vi "TcA01-007_ObjectsCanBeLookedUpByName.vi"(1 "Input buffer":T3="1", 3 "Invocation info":T2, 5 "error in (no error)":errorcluster, 6 "Add log to result?":bool) -> (16 "Test Data":T1 {"Numeric Measurement" format="%.2f"}, 19 "error out":errorcluster)   [LabVIEW 2020]
doc: "Test case template."
uses:
  Shared/Support_InputBuffer.ctl
  Shared/Support_InvocationInfo.ctl
  Shared/Support_TestData.ctl
  <vilib>/addons/_AddQ/G#Object/utils/G#Object_CreateMethod.ctl
  TestClasses/G#BaseClass1_class/G#BaseClass1.lvclass
  TestClasses/G#SubClass1_class/G#SubClass1.lvclass
  <vilib>/addons/_AddQ/G#Object/G#Object.lvclass
panel:
  in  "Test name":string="TcA01-007 Objects can be looked up by name"
  out "Test result":bool
  out "Result":string
  # "Verify that objects can be looked up by name and\nreturn that objects reference instead."
  # "Sub test case"
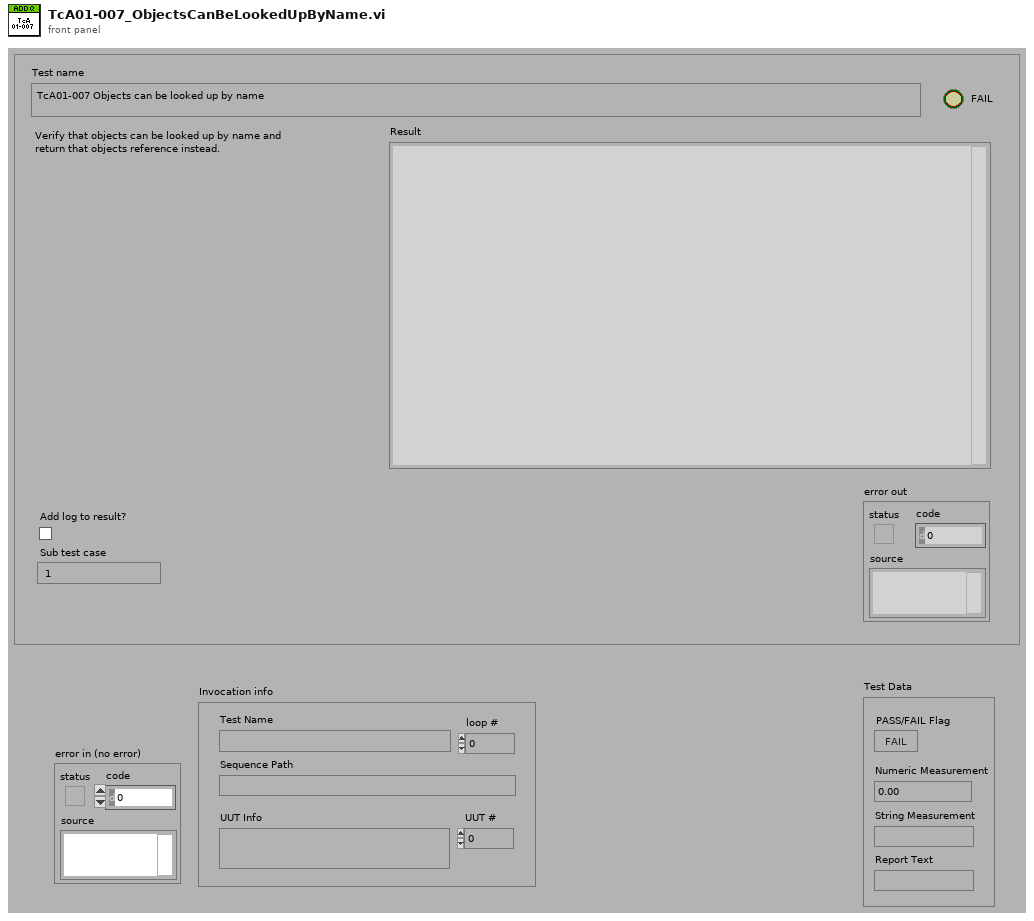
[diagram p1: front panel]
types:
  T1 = typedef "Support_TestData.ctl" = cluster{"PASS/FAIL Flag":bool, "Numeric Measurement":dbl, "String Measurement":string, "Report Text":string}
  T2 = typedef "Support_InvocationInfo.ctl" = cluster{"UUT #":i32, "loop #":i32, "UUT Info":string, "Test Name":string, "Sequence Path":path}
  T3 = typedef "Support_InputBuffer.ctl" = string
  T4 = typedef "G#Object.lvclass/G#Object_CreateMethod.ctl" = enum16{"Create", "Create or look up existing", "Look up existing"}
  T5 = typedef "Support_ResultType.ctl" = cluster{"Pass":bool, "Comment":string, "MeasurementValue":dbl}
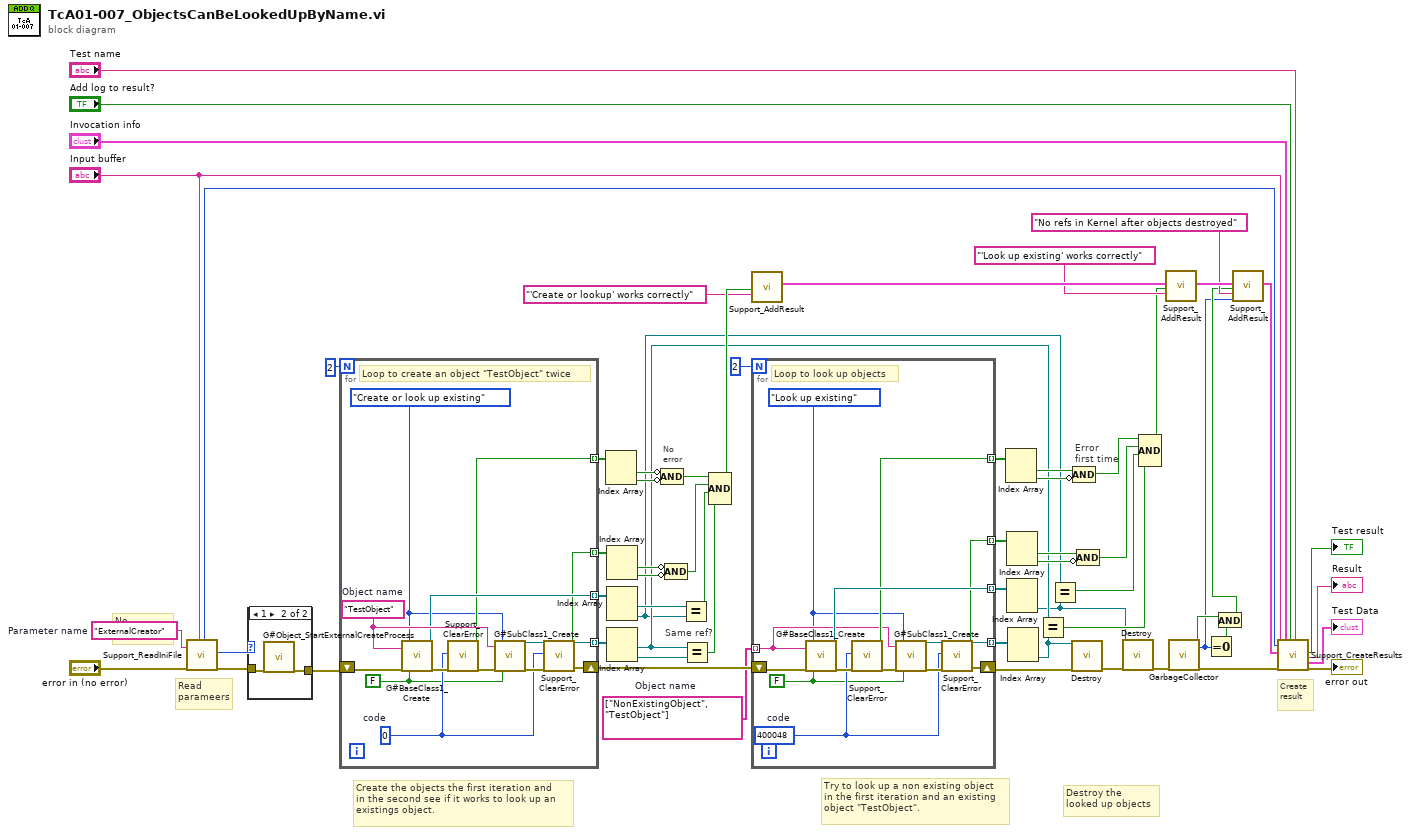
[diagram p0: block diagram]
diagram:
  w3 = "ExternalCreator"  # Parameter name
  w30 = string[] ["NonExistingObject", "TestObject"]  # Object name
  # "Create the objects the first iteration and\nin the second see if it works to look up an\nexistings object."
  # "Try to look up a non existing object\nin the first iteration and an existing\nobject \"TestObject\"."
  # "Destroy the\nlooked up objects"
  # "Error\nfirst time"
  # "Same ref?"
  # "No\nerror"
  # "No\nparameters"
  # "Create\nresult"
  # "Read\nparameers"
  n1 = call "Support_ReadIniFile.vi"("Parameter name"=w3, "error in (no error)"="error in (no error)", "Sub test case"="Input buffer") -> ("Timer start"=w55:u32, "Parameter1 as I32"=w5:i32, "error out"=w6:errorcluster)  [unwired: 9 in, 5 out]
  n2 = case shown="1" w5 {
    tunnel: w6 -> [w65 w67]
    tunnel: [w65 w66] -> w4
    frame 0, Default {
    }
    frame 1 {
      n3 = call <vilib>:"G#Object_StartExternalCreateProcess.vi"("error in (no error)"=w67) -> ("error out"=w66:errorcluster)  [unwired: 18 in]
    }
  }
  n4 = for {
    N: 2 -> [_]
    shift-right: [w72] -> w32
    shift-left: w4 -> [w77]
    tunnel: [w75] -> w51 mode=indexing
    tunnel: [w74] -> w50 mode=indexing
    tunnel: [w71] -> w53 mode=indexing
    tunnel: [w70] -> w52 mode=indexing
    w68 = FALSE ("user counter")
    w69 = G#Object_CreateMethod."Create or look up existing" ("create method")
    w73 = 0  # code
    w76 = "TestObject"  # Object name
    # "Loop to create an object \"TestObject\" twice"
    n5 = call "G#BaseClass1_Create.vi"("object name"=w76, "error in (no error)"=w77, "create method"=w69, "user counter"=w68) -> ("reference out"=w75:refnum<class "G#BaseClass1.lvclass">, "error out"=w78:errorcluster)  [unwired: 13 in, 1 out]
    n6 = call "Support_ClearError.vi"("code"=w73, "error in (no error)"=w78) -> ("Cleared?"=w71:bool, "error out"=w79:errorcluster)  [unwired: 16 in]
    n7 = call "G#SubClass1_Create.vi"("object name"=w76, "error in (no error)"=w79, "create method"=w69, "user counter"=w68) -> ("reference out"=w74:refnum<class "G#SubClass1.lvclass">, "error out"=w80:errorcluster)  [unwired: 13 in, 1 out]
    n8 = call "Support_ClearError.vi"("code"=w73, "error in (no error)"=w80) -> ("Cleared?"=w70:bool, "error out"=w72:errorcluster)  [unwired: 16 in]
  }
  n9 = Index Array(array=w53) -> (element #1=w47:bool, element #2=w46:bool)  [unwired: 2 in]
  n10 = Index Array(array=w52) -> (element #1=w45:bool, element #2=w44:bool)  [unwired: 2 in]
  n11 = Index Array(array=w51) -> (element #1=w49:refnum<class "G#BaseClass1.lvclass">, element #2=w2:refnum<class "G#BaseClass1.lvclass">)  [unwired: 2 in]
  n12 = Index Array(array=w50) -> (element #1=w13:refnum<class "G#SubClass1.lvclass">, element #2=w48:refnum<class "G#SubClass1.lvclass">)  [unwired: 2 in]
  n13 = Compound Arithmetic op=AND(invert w47, invert w46) -> (w43:bool)
  n14 = Compound Arithmetic op=AND(invert w45, invert w44) -> (w42:bool)
  n15 = Equal?(x=w49, y=w2) -> (x = y?=w41:bool)
  n16 = Equal?(x=w13, y=w48) -> (x = y?=w40:bool)
  n17 = Compound Arithmetic op=AND(w43, w42, w41, w40) -> (w39:bool)
  n18 = call "Support_AddResult.vi"("Pass"=w39, "Comment"="'Create or lookup' works correctly") -> ("Results out"=w37:T5[])  [unwired: 17 in]
  n19 = for {
    N: 2 -> [_]
    shift-right: [w86] -> w27
    shift-left: w32 -> [w90]
    tunnel: [w89] -> w25 mode=indexing
    tunnel: [w88] -> w26 mode=indexing
    tunnel: [w85] -> w19 mode=indexing
    tunnel: [w84] -> w20 mode=indexing
    tunnel: w30 -> [w83] mode=indexing
    w81 = FALSE ("user counter")
    w82 = G#Object_CreateMethod."Look up existing" ("create method")
    w87 = 400048  # code
    # "Loop to look up objects"
    n20 = call "G#BaseClass1_Create.vi"("object name"=w83, "error in (no error)"=w90, "create method"=w82, "user counter"=w81) -> ("reference out"=w89:refnum<class "G#BaseClass1.lvclass">, "error out"=w91:errorcluster)  [unwired: 13 in, 1 out]
    n21 = call "Support_ClearError.vi"("code"=w87, "error in (no error)"=w91) -> ("Cleared?"=w85:bool, "error out"=w92:errorcluster)  [unwired: 16 in]
    n22 = call "G#SubClass1_Create.vi"("object name"=w83, "error in (no error)"=w92, "create method"=w82, "user counter"=w81) -> ("reference out"=w88:refnum<class "G#SubClass1.lvclass">, "error out"=w93:errorcluster)  [unwired: 13 in, 1 out]
    n23 = call "Support_ClearError.vi"("code"=w87, "error in (no error)"=w93) -> ("Cleared?"=w84:bool, "error out"=w86:errorcluster)  [unwired: 16 in]
  }
  n24 = Index Array(array=w19) -> (element #1=w21:bool, element #2=w22:bool)  [unwired: 2 in]
  n25 = Index Array(array=w20) -> (element #1=w23:bool, element #2=w24:bool)  [unwired: 2 in]
  n26 = Index Array(array=w25) -> (element #2=w1:refnum<class "G#BaseClass1.lvclass">)  [unwired: 2 in, 1 out]
  n27 = Index Array(array=w26) -> (element #2=w14:refnum<class "G#SubClass1.lvclass">)  [unwired: 2 in, 1 out]
  n28 = Equal?(x=w13, y=w14) -> (x = y?=w11:bool)
  n29 = Equal?(x=w2, y=w1) -> (x = y?=w12:bool)
  n30 = call-dynamic "Destroy.vi"("reference in"=w14, "error in (no error)"=w27) -> ("error out"=w28:errorcluster)  [unwired: 16 in, 1 out]
  n31 = Compound Arithmetic op=AND(w21, invert w22) -> (w18:bool)
  n32 = Compound Arithmetic op=AND(w23, invert w24) -> (w17:bool)
  n33 = call-dynamic "Destroy.vi"("reference in"=w1, "error in (no error)"=w28) -> ("error out"=w29:errorcluster)  [unwired: 16 in, 1 out]
  n34 = Compound Arithmetic op=AND(w18, w17, w12, w11) -> (w16:bool)
  n35 = call "Support_AddResult.vi"("Results in"=w37, "Pass"=w16, "Comment"="'Look up existing' works correctly") -> ("Results out"=w36:T5[])  [unwired: 16 in]
  n36 = call <vilib>:"GarbageCollector.vi"("error in (no error)"=w29) -> ("OK"=w9:bool, "# of objects killed"=w7:i32, "error out"=w33:errorcluster)  [unwired: 16 in]
  n37 = Equal To 0?(x=w7) -> (x = 0?=w10:bool)
  n38 = And(x=w9, y=w10) -> (x .and. y?=w8:bool)
  n39 = call "Support_AddResult.vi"("Results in"=w36, "Pass"=w8, "Comment"="No refs in Kernel after objects destroyed", "MeasurementValue"=w7) -> ("Results out"=w35:T5[])  [unwired: 15 in]
  n40 = call "Support_CreateResults.vi"("Sub test case"="Input buffer", "Timer start"=w55, "Results"=w35, "error in (no error)"=w33, "Invocation info"="Invocation info", "Add log to result?"="Add log to result?", "Test name"="Test name") -> ("Pass/fail flag"=→"Test result":bool, "Result"=→"Result":string, "Test Data"=→"Test Data":T1, "error out"=→"error out":errorcluster)  [unwired: 9 in]
